vi "Open Deployed Stimulus Profile Session.vi"(8 "error in (no error)":errorcluster, 9 "Gateway IP Address (\"\": localhost)":string, 11 "Deployed Session ID":string) -> (0 "error out":errorcluster, 3 "Session Ref":T1)   [LabVIEW 2020, in "NI_VS Sequence Execution Interface.lvlib"]
doc: "Opens a reference to an existing stimulus profile session that has already been deployed."
uses:
  <vilib>/NI VeriStand/Execution/SequenceExecutionInterface/NI_VS Sequence Execution Interface.lvlib
  <vilib>/NI VeriStand/Execution/SequenceExecutionInterface/Stimulus Profile Session Ref.ctl
  NationalInstruments.VeriStand.ClientAPI
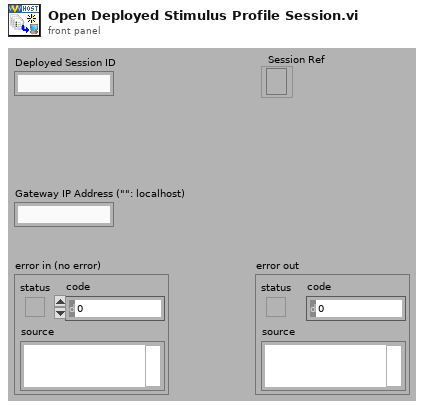
[diagram p1: front panel]
types:
  T1 = typedef "NI_VS Sequence Execution Interface.lvlib/Stimulus Profile Session Ref.ctl" = refnum<k24>
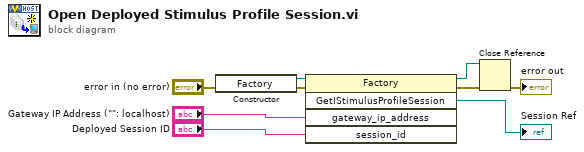
[diagram p0: block diagram]
diagram:
  n1 = constructor class="Factory"(error in="error in (no error)") -> (reference out=w8:refnum<k24>, error out=w9:errorcluster)  [unwired: 2 in, 1 out]
  n2 = invoke class="Factory" method="GetIStimulusProfileSession"(reference=w8, error in=w9, "gateway_ip_address"="Gateway IP Address (\"\": localhost)", "session_id"="Deployed Session ID") -> (reference out=w2:refnum<k24>, error out=w3:errorcluster, "GetIStimulusProfileSession"=→"Session Ref":refnum<k24>)  [unwired: 1 in, 2 out]
  n3 = Close Reference(reference=w2, error in (no error)=w3) -> (error out=→"error out":errorcluster)
